vi "SendComplexCluster.vi"(8 "error in (no error)":errorcluster, 10 "In":T1, 11 "reference in":refnum<class "PerformanceTest.lvclass">) -> (0 "error out":errorcluster, 2 "Out":T1, 3 "reference out":refnum<class "PerformanceTest.lvclass">)   [LabVIEW 2018, in "PerformanceTest.lvclass"]
uses:
  PerformanceTest.lvclass
  ComplexData.ctl
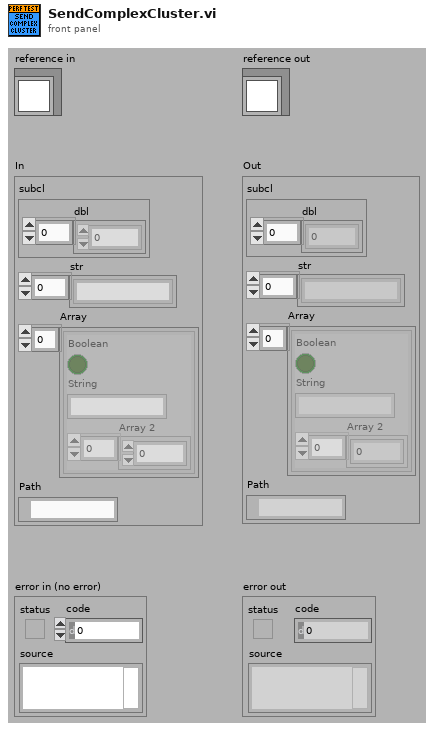
[diagram p1: front panel]
types:
  T1 = typedef "PerformanceTest.lvclass/ComplexData.ctl" = cluster{"subcl":cluster{"dbl":dbl[]}, "str":string[], "Array":cluster{"Boolean":bool, "String":string, "Array 2":dbl[]}[], "Path":path}
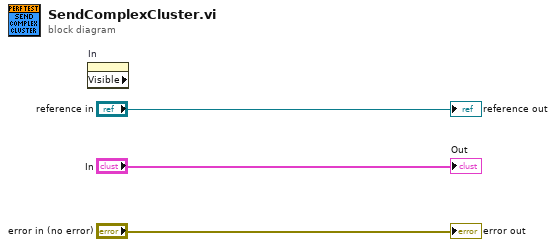
[diagram p0: block diagram]
diagram:
  n1 = property on="In" class="Clust (strict)" props=["Visible"]() -> ()  [unwired: 2 in, 3 out]
  "error out" <- "error in (no error)"
  "reference out" <- "reference in"
  "Out" <- "In"
